vi "StrToPW.vi"(8 "error in":errorcluster caption="错误输入", 11 "StrIn":string) -> (0 "error out":errorcluster caption="错误输出", 3 "StrOut":string)   [LabVIEW 2013]
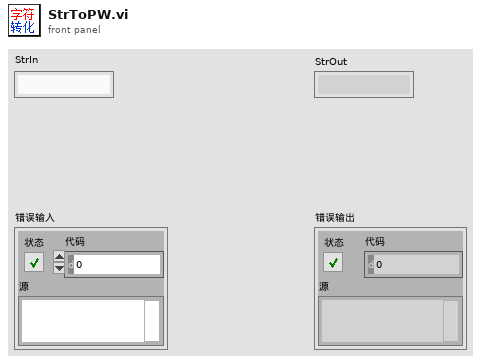
[diagram p1: front panel]
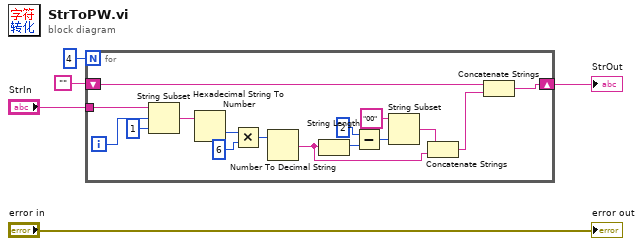
[diagram p0: block diagram]
diagram:
  n1 = for {
    N: 4 -> [_]
    tunnel: "StrIn" -> [w21]
    shift-right: [w6] -> w4
    shift-left: "" -> [w8]
    i -> [w20]
    n2 = String Subset(string=w21, offset (0)=w20, length (rest)=1 ("长度（剩余）")) -> (substring=w18:string)
    n3 = Hexadecimal String To Number(string=w18) -> (number=w17:u32)  [unwired: 2 in, 1 out]
    n4 = Multiply(x=w17, y=6) -> (x*y=w15:u32)
    n5 = Number To Decimal String(number=w15) -> (decimal integer string=w9:string)  [unwired: 1 in]
    n6 = String Length(string=w9) -> (length=w14:i32)
    n7 = Subtract(x=2, y=w14) -> (x-y=w12:i32)
    n8 = String Subset(string="00", length (rest)=w12) -> (substring=w10:string)  [unwired: 1 in]
    n9 = Concatenate Strings(w10, w9) -> (w7:string)
    n10 = Concatenate Strings(w8, w7) -> (w6:string)
  }
  "StrOut" <- w4
  "error out" <- "error in"
